vi "glopost.vi"() -> ()   [LabVIEW 2013]
panel:
  out "position":dbl
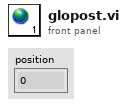
[diagram p1: front panel]
diagram:
